vi "GetAPSxParameter.vi"(8 "error in (no error)":errorcluster caption="错误输入（无错误）", 10 "Param":T1(ring), 11 "hASIC":i32) -> (0 "error out":errorcluster caption="错误输出", 3 "iPrevValue":i32)   [LabVIEW 2018]
doc: "该模板用于创建子VI。"
uses:
  APSx.dll/APSx.dll
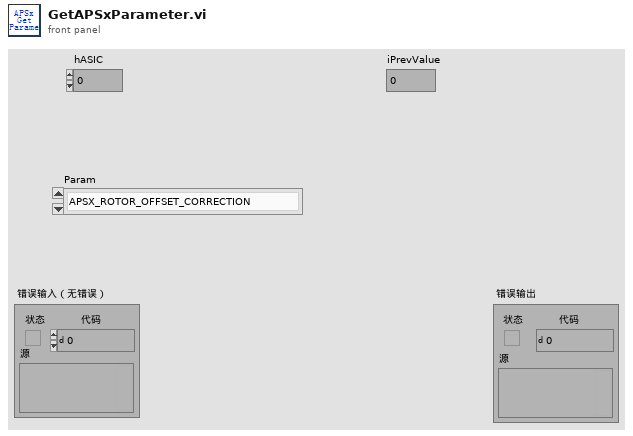
[diagram p1: front panel]
types:
  T1 = enum16{"APSX_ROTOR_OFFSET_CORRECTION", "APSX_SCALING"}
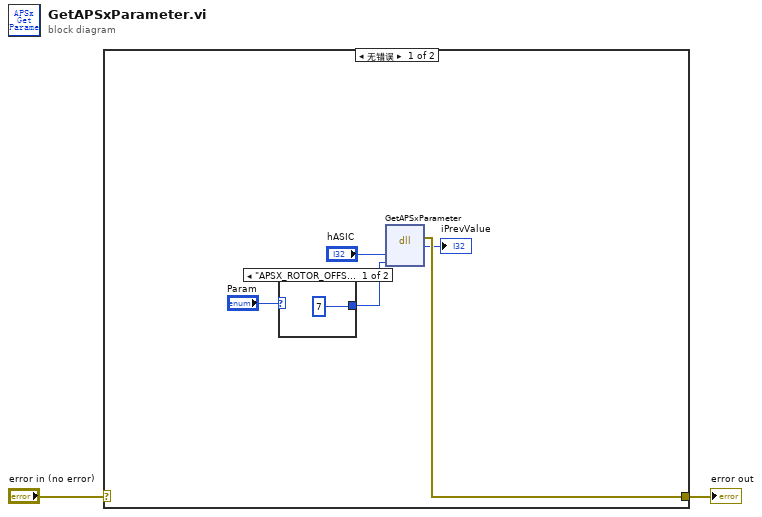
[diagram p0: block diagram]
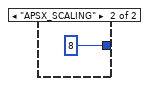
[diagram p2: hidden frame]
diagram:
  n1 = case shown="无错误" "error in (no error)" {
    selector: "error in (no error)" -> [_ w10]
    tunnel: [w7 w10] -> w1
    frame No Error {
      n2 = case shown="\"APSX_ROTOR_OFFSET_CORRECTION\", 默认" "Param" {
        tunnel: [7 8] -> w3
        frame "APSX_ROTOR_OFFSET_CORRECTION", Default {
        }
        frame "APSX_SCALING" {
        }
      }
      n3 = dll-call lib="PTH2]abs D项目Feng恒隆项目Labview传感器对中台SourcesAPSx.dllAPSx.dll" fn="GetAPSxParameter"("hASIC"="hASIC", "Param"=w3) -> (error out=w7:errorcluster, "iPrevValue"=→"iPrevValue":i32)  [unwired: 5 in, 1 out]
    }
    frame Error {
    }
  }
  "error out" <- w1
